vi "Snap from Camera (SubVI).vi"(6 "error in":errorcluster, 8 "Live":bool, 9 "Image Size in":T1={"Rows (X)"=256, "Colums (Y)"=256}, 10 "Session In":T2, 11 "Image in":T3) -> (0 "Image Pixels (U8)":u8[][](array[numeric]), 1 "Image Size out":T1={"Rows (X)"=256, "Colums (Y)"=256}, 2 "Session Out":T2, 3 "Image out":T3, 4 "error out":errorcluster)   [LabVIEW 2025, in "SoC IP Library.lvlib"]
uses:
  SoC IP Library.lvlib
  <vilib>/vision/Image Controls.llb/IMAQ Image.ctl
  <vilib>/userDefined/High Color/IMAQdx.ctl
  Controls/Image Size.ctl
  <vilib>/vision/driver/NI_Vision_Acquisition_Software.lvlib
  <vilib>/vision/NI_Vision_Development_Module.lvlib
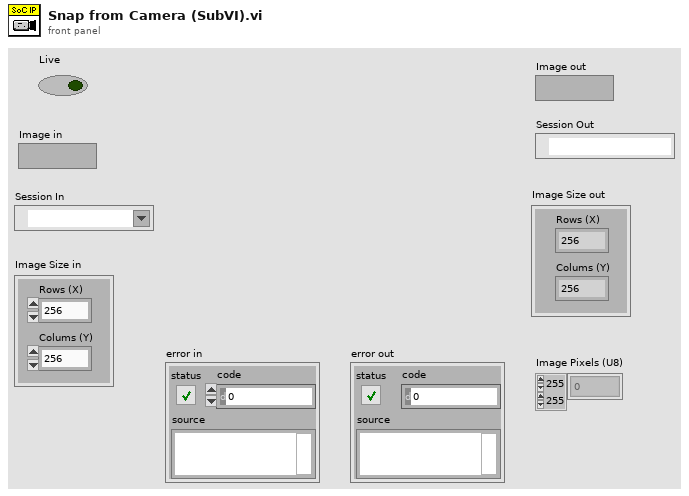
[diagram p1: front panel]
types:
  T1 = typedef "SoC IP Library.lvlib/Image Size.ctl" = cluster{"Rows (X)":u16, "Colums (Y)":u16}
  T2 = typedef "IMAQdx.ctl" = refnum<k21>
  T3 = typedef "IMAQ Image.ctl" = refnum<image>
  T4 = typedef "Image Type" = u32
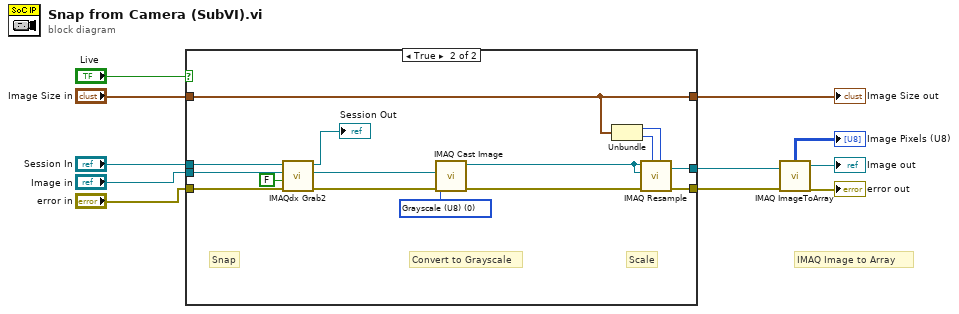
[diagram p0: block diagram]
diagram:
  # "IMAQ Image to Array"
  n1 = case shown="True" "Live" {
    tunnel: "Image in" -> [w11 w23]
    tunnel: "error in" -> [w13 w22]
    tunnel: [w13 w19] -> w5
    tunnel: "Image Size in" -> [w12 w16]
    tunnel: [w12 w16] -> w3
    tunnel: "Session In" -> [_ w15]
    tunnel: [w11 w14] -> w1
    frame False {
    }
    frame True {
      w26 = T4 0 items=["Grayscale (U8)", "Grayscale (I16)", "Grayscale (SGL)", "Complex (CSG)", "RGB (U32)", "HSL (U32)", "RGB (U64)", "Grayscale (U16)"] ("Image Type")
      # "Scale"
      # "Convert to Grayscale"
      # "Snap"
      n2 = call <vilib>:"IMAQdx Grab2.vi"("error in"=w22, "Wait for Next Buffer? (Yes)"=FALSE, "Image In"=w23, "Session In"=w15) -> ("error out"=w24:errorcluster, "Image Out"=w25:T3, "Session Out"=→"Session Out":T2)  [unwired: 4 in, 1 out]
      n3 = call "IMAQ Cast Image"("Image Type"=w26, "error in (no error)"=w24, "Image Dst"=w25, "Image Src"=w25) -> ("error out"=w27:errorcluster, "Image Dst Out"=w28:T3)  [unwired: 6 in]
      n4 = Unbundle(w16) -> ("Rows (X)"=w17:u16, "Colums (Y)"=w18:u16)
      n5 = call "IMAQ Resample"("X Resolution"=w17, "Y Resolution"=w18, "error in (no error)"=w27, "Image Dst"=w28, "Image Src"=w28) -> ("error out"=w19:errorcluster, "Image Dst Out"=w14:T3)  [unwired: 5 in]
    }
  }
  "Image out" <- w1
  "Image Size out" <- w3
  n6 = call "IMAQ ImageToArray"("error in (no error)"=w5, "Image"=w1) -> ("error out"=→"error out":errorcluster, "Image Pixels (U8)"=→"Image Pixels (U8)":u8[][])  [unwired: 2 in, 3 out]
